vi "ScopeConfigure.vi"(0 "VISA resource name":refnum<visa-resource-name>="USB0::0x1AB1::0x0488::DS1BA202100064::INSTR", 1 "scaleTime":dbl=0.0005 format="%#_6f", 3 "triggerVoltage":dbl=1.5, 4 "scaleVoltage":dbl=5.0, 5 "error in (no error)":errorcluster, 6 "Channel (0: Channel 1)":u16(ring) items=["Channel 1", "Channel 2", "Channel 3", "Channel 4"], 7 "Attenuation":i32=1, 8 "offsetVoltage":dbl format="%#_6f", 9 "offsetTime":dbl format="%#_6f", 10 "Vertical Coupling (0: DC)":u16(ring) items=["DC", "AC", "Ground"], 11 "Trigger Type (0: Edge)":u16(ring) items=["Edge", "Pulse", "Video", "Pattern", "Duration"], 12 "BW Selector":bool, 13 "F Selector":bool) -> (14 "VISA resource name out":refnum<visa-resource-name>, 19 "error out":errorcluster)   [LabVIEW 2018]
uses:
  <vilib>/Utility/error.llb/DialogType.ctl
  <instrlib>/RIGOL DS1000 Series/RIGOL DS1000 Series.lvlib
panel:
  out "offsetV":string
  out "offsetT":string
  out "Command sent":string
  out "chann":string
  out "attn":string
  out "scaleT":string
  out "scaleV":string
  out "band":string
  out "trigger":string
  out "filter":string
  # "Probe"
  # "Vertical"
  # "Horizontal"
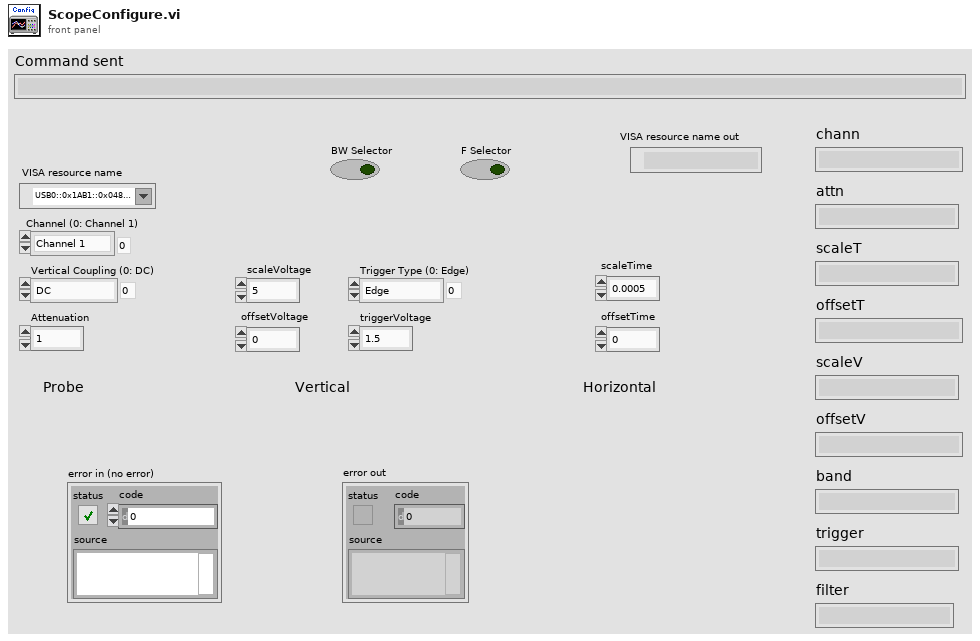
[diagram p1: front panel]
types:
  T1 = typedef "DialogType.ctl" = u16
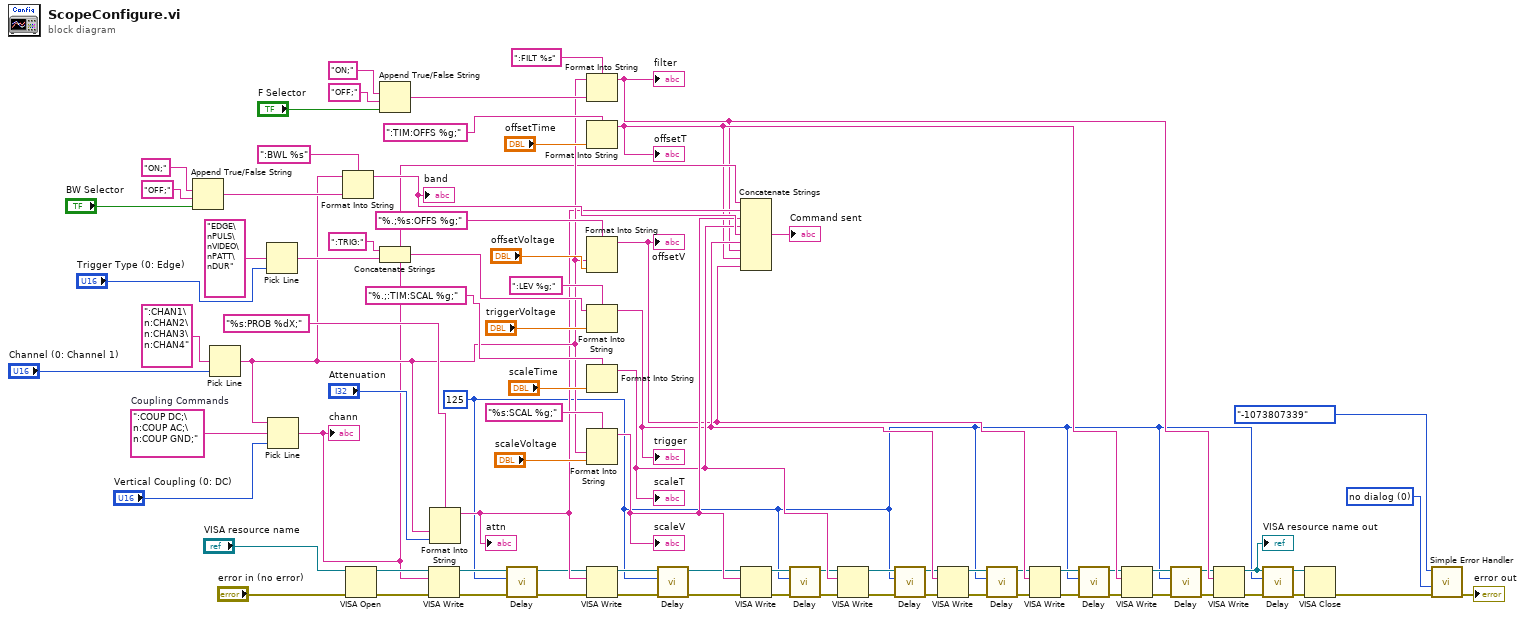
[diagram p0: block diagram]
diagram:
  w4 = u32 125 ("Delay (ms)")
  w50 = T1 0 items=["no dialog", "OK message", "continue or stop message", "OK message + warnings", "continue/stop + warnings"] ("type of dialog (OK msg:1)")
  w75 = ":COUP DC;\n:COUP AC;\n:COUP GND;"  # Coupling Commands
  n1 = Append True/False String(1:"BW Selector", 2:"OFF;" ("false string"), 3:"ON;" ("true string")) -> (0:w72:string)  [unwired: 1 out]
  n2 = Pick Line(multi-line string=":CHAN1\n:CHAN2\n:CHAN3\n:CHAN4" ("多行字符串"), line index="Channel (0: Channel 1)") -> (output string=w43:string)  [unwired: 1 out]
  n3 = Pick Line(multi-line string="EDGE\nPULS\nVIDEO\nPATT\nDUR", line index="Trigger Type (0: Edge)") -> (output string=w68:string)  [unwired: 1 out]
  n4 = Pick Line(string ("")=w43, multi-line string=w75, line index="Vertical Coupling (0: DC)") -> (output string=w42:string)
  "chann" <- w42
  n5 = Format Into String(format string=":BWL %s", initial string=w43, w72) -> (resulting string=w55:string)  [unwired: 1 in, 1 out]
  "band" <- w55
  n6 = VISA Open(error in (no error)="error in (no error)", VISA resource name="VISA resource name") -> (VISA resource name=w53:refnum<visa-resource-name>, error out=w21:errorcluster)  [unwired: 3 in]
  n7 = Append True/False String(1:"F Selector", 2:"OFF;" ("false string"), 3:"ON;" ("true string")) -> (0:w58:string)  [unwired: 1 out]
  n8 = Concatenate Strings(":TRIG:" ("string (\"\")"), w68) -> (w62:string)
  n9 = VISA Write(VISA resource name=w53, write buffer=w42, error in (no error)=w21) -> (VISA resource name out=w22:refnum<visa-resource-name>, error out=w20:errorcluster)  [unwired: 1 out]
  n10 = Format Into String(format string="%s:PROB %dX;", w43, "Attenuation") -> (resulting string=w41:string)  [unwired: 2 in, 1 out]
  "attn" <- w41
  n11 = call <instrlib>:"Delay.vi"("error in (no error)"=w20, "Delay (ms)"=w4, "VISA resource name"=w22) -> ("error out"=w19:errorcluster, "VISA resource name out"=w5:refnum<visa-resource-name>)  [unwired: 7 in]
  n12 = Format Into String(format string=":FILT %s", initial string=w43, w58) -> (resulting string=w35:string)  [unwired: 1 in, 1 out]
  "filter" <- w35
  n13 = Format Into String(format string=":TIM:OFFS %g;", "offsetTime") -> (resulting string=w36:string)  [unwired: 2 in, 1 out]
  "offsetT" <- w36
  n14 = Format Into String(format string="%.;%s:OFFS %g;", w43, "offsetVoltage") -> (resulting string=w37:string)  [unwired: 2 in, 1 out]
  "offsetV" <- w37
  n15 = Format Into String(format string=":LEV %g;", initial string=w62, "triggerVoltage") -> (resulting string=w38:string)  [unwired: 1 in, 1 out]
  "trigger" <- w38
  n16 = Format Into String(format string="%.;:TIM:SCAL %g;", "scaleTime") -> (resulting string=w39:string)  [unwired: 2 in, 1 out]
  "scaleT" <- w39
  n17 = Format Into String(format string="%s:SCAL %g;", w43, "scaleVoltage") -> (resulting string=w40:string)  [unwired: 2 in, 1 out]
  "scaleV" <- w40
  n18 = VISA Write(VISA resource name=w5, write buffer=w41, error in (no error)=w19) -> (VISA resource name out=w23:refnum<visa-resource-name>, error out=w18:errorcluster)  [unwired: 1 out]
  n19 = call <instrlib>:"Delay.vi"("error in (no error)"=w18, "Delay (ms)"=w4, "VISA resource name"=w23) -> ("error out"=w17:errorcluster, "VISA resource name out"=w24:refnum<visa-resource-name>)  [unwired: 7 in]
  n20 = Concatenate Strings(w42, w41, w40, w39, w55, w38, w35, w36, w37) -> (→"Command sent":string)
  n21 = VISA Write(VISA resource name=w24, write buffer=w40, error in (no error)=w17) -> (VISA resource name out=w25:refnum<visa-resource-name>, error out=w16:errorcluster)  [unwired: 1 out]
  n22 = call <instrlib>:"Delay.vi"("error in (no error)"=w16, "Delay (ms)"=w4, "VISA resource name"=w25) -> ("error out"=w15:errorcluster, "VISA resource name out"=w26:refnum<visa-resource-name>)  [unwired: 7 in]
  n23 = VISA Write(VISA resource name=w26, write buffer=w39, error in (no error)=w15) -> (VISA resource name out=w27:refnum<visa-resource-name>, error out=w14:errorcluster)  [unwired: 1 out]
  n24 = call <instrlib>:"Delay.vi"("error in (no error)"=w14, "Delay (ms)"=w4, "VISA resource name"=w27) -> ("error out"=w13:errorcluster, "VISA resource name out"=w28:refnum<visa-resource-name>)  [unwired: 7 in]
  n25 = VISA Write(VISA resource name=w28, write buffer=w38, error in (no error)=w13) -> (VISA resource name out=w29:refnum<visa-resource-name>, error out=w12:errorcluster)  [unwired: 1 out]
  n26 = call <instrlib>:"Delay.vi"("error in (no error)"=w12, "Delay (ms)"=w4, "VISA resource name"=w29) -> ("error out"=w11:errorcluster, "VISA resource name out"=w30:refnum<visa-resource-name>)  [unwired: 7 in]
  n27 = VISA Write(VISA resource name=w30, write buffer=w37, error in (no error)=w11) -> (VISA resource name out=w31:refnum<visa-resource-name>, error out=w10:errorcluster)  [unwired: 1 out]
  n28 = call <instrlib>:"Delay.vi"("error in (no error)"=w10, "Delay (ms)"=w4, "VISA resource name"=w31) -> ("error out"=w9:errorcluster, "VISA resource name out"=w32:refnum<visa-resource-name>)  [unwired: 7 in]
  n29 = VISA Write(VISA resource name=w32, write buffer=w36, error in (no error)=w9) -> (VISA resource name out=w33:refnum<visa-resource-name>, error out=w8:errorcluster)  [unwired: 1 out]
  n30 = call <instrlib>:"Delay.vi"("error in (no error)"=w8, "Delay (ms)"=w4, "VISA resource name"=w33) -> ("error out"=w7:errorcluster, "VISA resource name out"=w34:refnum<visa-resource-name>)  [unwired: 7 in]
  n31 = VISA Write(VISA resource name=w34, write buffer=w35, error in (no error)=w7) -> (VISA resource name out=w6:refnum<visa-resource-name>, error out=w3:errorcluster)  [unwired: 1 out]
  "VISA resource name out" <- w6
  n32 = call <instrlib>:"Delay.vi"("error in (no error)"=w3, "Delay (ms)"=w4, "VISA resource name"=w6) -> ("error out"=w51:errorcluster, "VISA resource name out"=w52:refnum<visa-resource-name>)  [unwired: 7 in]
  n33 = VISA Close(VISA resource name=w52, error in (no error)=w51) -> (error out=w48:errorcluster)
  n34 = call <vilib>:"Simple Error Handler.vi"("error code (no error:0)"=enum16{"-1073807339"}."-1073807339", "type of dialog (OK msg:1)"=w50, "error in (no error)"=w48) -> ("error out"=→"error out":errorcluster)  [unwired: 2 in, 4 out]
